vi "Initial Status Read.vi"(8 "error in (no error)":errorcluster, 11 "IgusMotorDrive in":refnum<class "IgusMotorDrive.lvclass">) -> (0 "error out":errorcluster, 1 "Response":T1={"Function Code"=1, "Data"=[], "RTU_DataBytes"=0} {"Data" format="%.0x"}, 2 "Command":T1={"Function Code"=1, "Data"=[], "RTU_DataBytes"=0} {"Data" format="%.0x"}, 3 "IgusMotorDrive out":refnum<class "IgusMotorDrive.lvclass">, 4 "Statusword":T2, 5 "Statusword out":T3)   [LabVIEW 2016, in "IgusMotorDrive.lvclass"]
doc: "Reads the status word from the drive\n\n<b>Copyright (C) 2018 Control Software Solutions Limited. All rights reserved. </b>"
uses:
  IgusMotorDrive.lvclass
  typedefs/Statusword--enum.ctl
  typedefs/Statusword--cluster.ctl
  Libraries/Modbus-Master/MB Master.lvlib
  Libraries/Modbus-Master/MB_Master_TCP/MB_Master_TCP.lvclass
  Libraries/Modbus-Master/MB_PDU/MB_PDU_Cluster.ctl
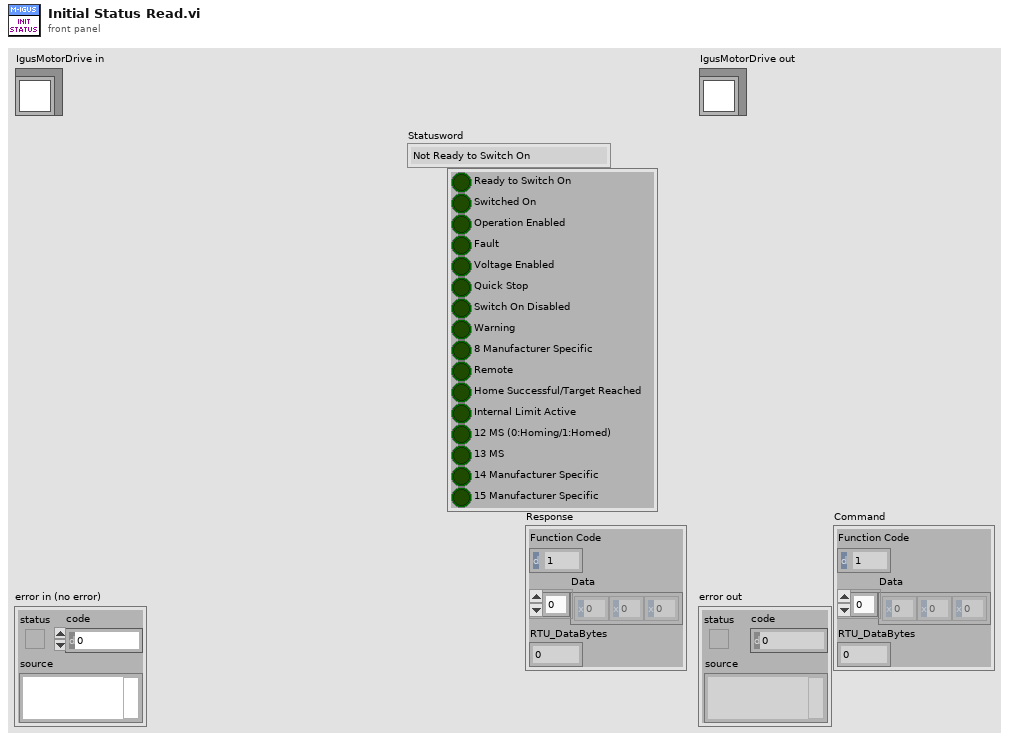
[diagram p1: front panel]
types:
  T1 = typedef "MB Master.lvlib/MB_PDU_Cluster.ctl" = cluster{"Function Code":u8, "Data":u8[], "RTU_DataBytes":i32}
  T2 = typedef "IgusMotorDrive.lvclass/Statusword--enum.ctl" = enum16{"Not Ready to Switch On", "Switch On Disabled", "Ready to Switch On", "Switched On", "Operation Enabled", "Quick Stop Active", "Fault Reaction Active", "Fault", "<Unknown>"}
  T3 = typedef "IgusMotorDrive.lvclass/Statusword--cluster.ctl" = cluster{"Ready to Switch On":bool, "Switched On":bool, "Operation Enabled":bool, "Fault":bool, "Voltage Enabled":bool, "Quick Stop":bool, "Switch On Disabled":bool, "Warning":bool, "8 Manufacturer Specific":bool, "Remote":bool, "Home Successful/Target Reached":bool, "Internal Limit Active":bool, "12 MS (0:Homing/1:Homed)":bool, "13 MS":bool, "14 Manufacturer Specific":bool, "15 Manufacturer Specific":bool}
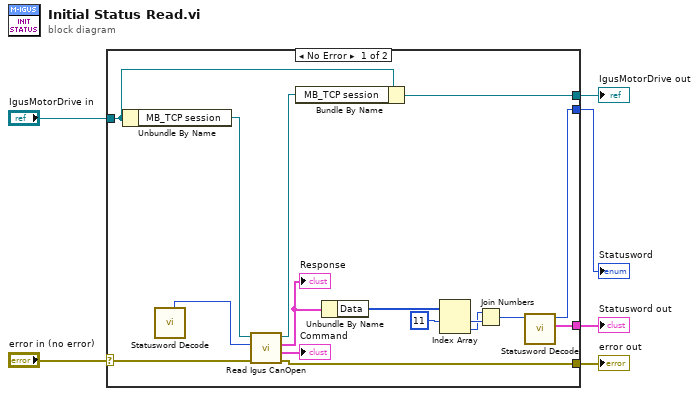
[diagram p0: block diagram]
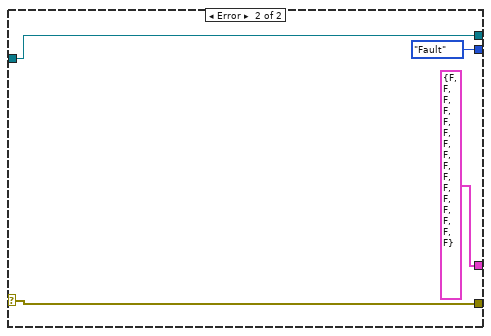
[diagram p2: hidden frame]
diagram:
  n1 = case shown="No Error" "error in (no error)" {
    selector: "error in (no error)" -> [w19 w26]
    tunnel: [w18 w26] -> w5
    tunnel: [w21 w25] -> w3
    tunnel: "IgusMotorDrive in" -> [w22 w25]
    tunnel: [w15 T3 {"Ready to Switch On"=FALSE, "Switched On"=FALSE, "Operation Enabled"=FALSE, "Fault"=FALSE, "Voltage Enabled"=FALSE, "Quick Stop"=FALSE, "Switch On Disabled"=FALSE, "Warning"=FALSE, "8 Manufacturer Specific"=FALSE, "Remote"=FALSE, "Home Successful/Target Reached"=FALSE, "Internal Limit Active"=FALSE, "12 MS (0:Homing/1:Homed)"=FALSE, "13 MS"=FALSE, "14 Manufacturer Specific"=FALSE, "15 Manufacturer Specific"=FALSE} ("Statusword out")] -> w2
    tunnel: [w14 Statusword--enum."Fault" ("Statusword")] -> w1
    frame No Error {
      n2 = Unbundle By Name(w22) -> ("MB_TCP session"=w17:refnum<class "MB_Master_TCP.lvclass">)
      n3 = call "Statusword Decode.vi"() -> ("address"=w20:u16)  [unwired: 8 in, 3 out]
      n4 = call "Read Igus CanOpen.vi"("error in (no error)"=w19, "Address"=w20, "MB session in"=w17) -> ("error out"=w18:errorcluster, "Command"=→"Command":T1, "Response"=w9:T1, "MB session out"=w16:refnum<class "MB_Master_TCP.lvclass">)  [unwired: 5 in]
      "Response" <- w9
      n5 = Bundle By Name(cluster=w22, "MB_TCP session"=w16) -> (w21:refnum<class "IgusMotorDrive.lvclass">)
      n6 = Unbundle By Name(w9) -> ("Data"=w13:u8[])
      n7 = Index Array(array=w13, index #1=11 ("index")) -> (element #1=w11:u8, element #2=w10:u8)  [unwired: 1 in]
      n8 = Join Numbers(hi=w10, lo=w11) -> ((hi.lo)=w8:u16)
      n9 = call "Statusword Decode.vi"("Statusword U16"=w8) -> ("Statusword out"=w15:T3, "Statusword"=w14:T2)  [unwired: 7 in, 2 out]
    }
    frame Error {
    }
  }
  "error out" <- w5
  "IgusMotorDrive out" <- w3
  "Statusword out" <- w2
  "Statusword" <- w1
